vi "Mean_fr_NaN_data.vi"(0 "Data":dbl[](array[numeric]) format="%.2f") -> (1 "Mean value":dbl format="%.2f", 2 "GoodFraction":dbl)   [LabVIEW 2022 SP3]
uses:
  <vilib>/Analysis/baseanly.llb/Mean (DBL).vi
  <vilib>/Analysis/NI_AALBase.lvlib
panel:
  # "Removes NaNs from array and computes mean of remaining samples.\nIf GoodFraction <0.5 will still report NaN."
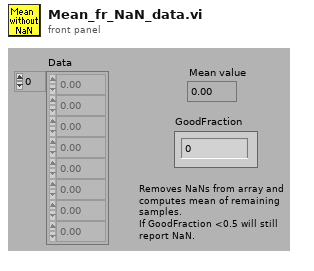
[diagram p1: front panel]
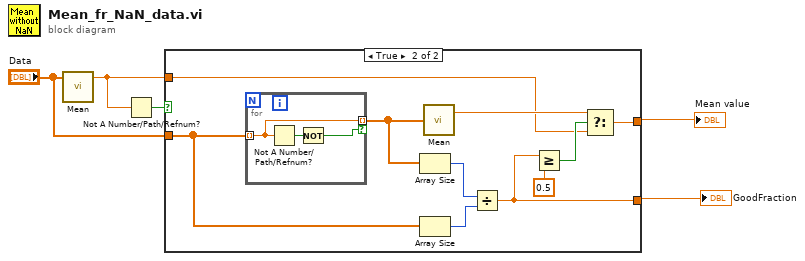
[diagram p0: block diagram]
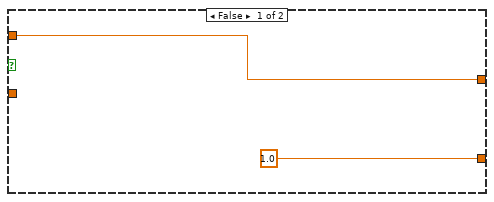
[diagram p2: hidden frame]
diagram:
  n1 = call-poly <vilib>:"Mean.vi"("X"="Data") -> ("mean"=w3:dbl)  [unwired: 1 out]
  n2 = Not A Number/Path/Refnum?(number/path/refnum=w3) -> (NaN/Path/Refnum?=w2:bool)
  n3 = case shown="True" w2 {
    tunnel: "Data" -> [_ w17]
    tunnel: [w7 w8] -> w4
    tunnel: w3 -> [w7 w9]
    tunnel: [1.0 w13] -> w1
    frame False {
    }
    frame True {
      n4 = for {
        tunnel: w17 -> [w19] mode=indexing
        tunnel: [w19] -> w14 mode=indexing if=w18
        n5 = Not A Number/Path/Refnum?(number/path/refnum=w19) -> (NaN/Path/Refnum?=w20:bool)
        n6 = Not(x=w20) -> (.not. x?=w18:bool)
      }
      n7 = Array Size(array=w14) -> (size(s)=w16:i32)
      n8 = Array Size(array=w17) -> (size(s)=w15:i32)
      n9 = call-poly <vilib>:"Mean.vi"("X"=w14) -> ("mean"=w10:dbl)  [unwired: 1 out]
      n10 = Divide(x=w16, y=w15) -> (x/y=w13:dbl)
      n11 = Greater Or Equal?(x=w13, y=0.5) -> (x >= y?=w11:bool)
      n12 = Select(t=w10, s=w11, f=w9) -> (s? t:f=w8:dbl)
    }
  }
  "Mean value" <- w4
  "GoodFraction" <- w1
